vi "Snap to Grid.vi"(8 "error in (no error)":errorcluster, 11 "VI Refnum in":refnum<vi>) -> (0 "error out":errorcluster, 3 "VI Refnum out":refnum<vi>)   [LabVIEW 2019, in "Builtins.lvlib"]
doc: "Snaps the selected front panel controls to the nearest VI panel grid size. If nothing is selected, this snaps all panel controls to grid. Default grid size is 12px.\n\nCreated by: Ryan Pacini"
uses:
  Builtins.lvlib
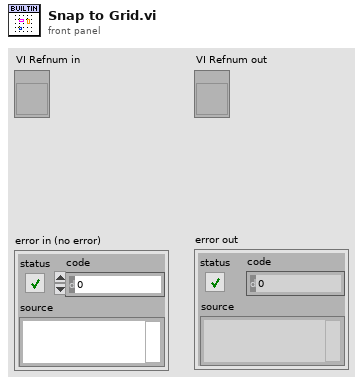
[diagram p1: front panel]
types:
  T1 = typedef "LVRectTypeDef.ctl" = cluster{"Left":i16, "Top":i16, "Right":i16, "Bottom":i16}
  T2 = cluster{"Left":i16, "Top":i16, "Right":i16, "Bottom":i16}[]
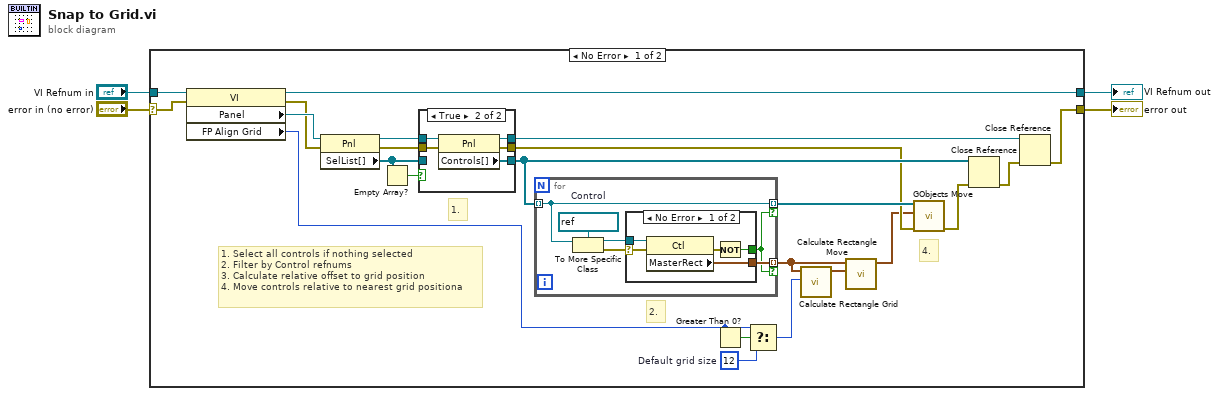
[diagram p0: block diagram]
diagram:
  n1 = case shown="No Error" "error in (no error)" {
    selector: "error in (no error)" -> [w25 w47]
    tunnel: "VI Refnum in" -> [w23 w48]
    tunnel: [w27 w48] -> w3
    tunnel: [w26 w47] -> w2
    frame No Error {
      w10 = 12  # Default grid size
      # "4."
      # "2."
      # "1."
      # "1. Select all controls if nothing selected\n2. Filter by Control refnums\n3. Calculate relative offset to grid position\n4. Move controls relative to nearest grid positiona"
      n2 = property class="VI"(reference=w23, error in=w25) -> (reference out=w27:refnum<vi>, error out=w22:errorcluster, "Panel"=w24:refnum<vi>, "FP Align Grid"=w9:i32)
      n3 = property class="Pnl"(reference=w24, error in=w22) -> (reference out=w21:refnum<vi>, error out=w18:errorcluster, "SelList[]"=w17:refnum<vi>[])
      n4 = Empty Array?(array=w17) -> (empty?=w16:bool)
      n5 = case shown="True" w16 {
        tunnel: w21 -> [w28 w35]
        tunnel: [w28 w34] -> w19
        tunnel: w18 -> [w29 w33]
        tunnel: w17 -> [w30 _]
        tunnel: [w29 w32] -> w12
        tunnel: [w30 w31] -> w15
        frame False {
        }
        frame True {
          n6 = property class="Pnl"(reference=w35, error in=w33) -> (reference out=w34:refnum<vi>, error out=w32:errorcluster, "Controls[]"=w31:refnum<vi>[])
        }
      }
      n7 = for {
        tunnel: w15 -> [w39] mode=indexing
        tunnel: [w39] -> w13 mode=indexing if=w36
        tunnel: [w37] -> w7 mode=indexing if=w36
        w41 = refnum<vi> refnum  # Control
        n8 = To More Specific Class(target class=w41, reference=w39) -> (specific class reference=w38:refnum<vi>, error out=w40:errorcluster)  [unwired: 1 in]
        n9 = case shown="No Error" w40 {
          selector: w40 -> [w46 _]
          tunnel: w38 -> [w44 _]
          tunnel: [w43 _] -> w37
          tunnel: [w42 _] -> w36
          frame No Error {
            n10 = property class="Ctl"(reference=w44, error in=w46) -> (error out=w45:errorcluster, "MasterRect"=w43:T1)  [unwired: 1 out]
            n11 = Not(x=w45) -> (.not. x?=w42:bool)
          }
          frame Error {
          }
        }
      }
      n12 = Greater Than 0?(x=w9) -> (x > 0?=w11:bool)
      n13 = Select(t=w9, s=w11, f=w10) -> (s? t:f=w8:i32)
      n14 = call "Calculate Rectangle Grid.vi"("Grid Size (12px)"=w8, "Rects in"=w7) -> ("Resolved Rects out"=w6:T2)  [unwired: 9 in]
      n15 = call "Calculate Rectangle Move.vi"("End Rects out"=w6, "Start Rects in"=w7) -> ("Relative Move"=w5:cluster{"Left":i32, "Top":i32}[])  [unwired: 9 in]
      n16 = call "GObjects Move.vi"("error in (no error)"=w12, "Relative Moves in"=w5, "GObjects in"=w13) -> ("error out"=w14:errorcluster)  [unwired: 7 in, 1 out]
      n17 = Close Reference(reference=w15, error in (no error)=w14) -> (error out=w20:errorcluster)
      n18 = Close Reference(reference=w19, error in (no error)=w20) -> (error out=w26:errorcluster)
    }
    frame Error {
    }
  }
  "VI Refnum out" <- w3
  "error out" <- w2
